vi "Stop Data Logging Session.vi"(8 "error in (no error)":errorcluster, 9 "Clear Session (T)":bool=TRUE, 10 "Session Name in":string, 11 "Data Logging Manager Ref in":T1) -> (0 "error out":errorcluster, 1 "Log File Paths":path[](array[path]), 2 "Session Name out":string, 3 "Data Logging Manager Ref out":T1)   [LabVIEW 2020, in "NI_VS Data Logging API.lvlib"]
doc: "Stops the data logging session specified by <B>Session Name in</B> and returns the paths to all log files generated during the session. This VI attempts to stop the data logging session regardless of any incoming errors."
uses:
  <vilib>/NI VeriStand/Execution/DataLogging/NI_VS Data Logging API.lvlib
  <vilib>/NI VeriStand/Execution/DataLogging/IDataLogging Ref.ctl
  NationalInstruments.VeriStand.ClientAPI
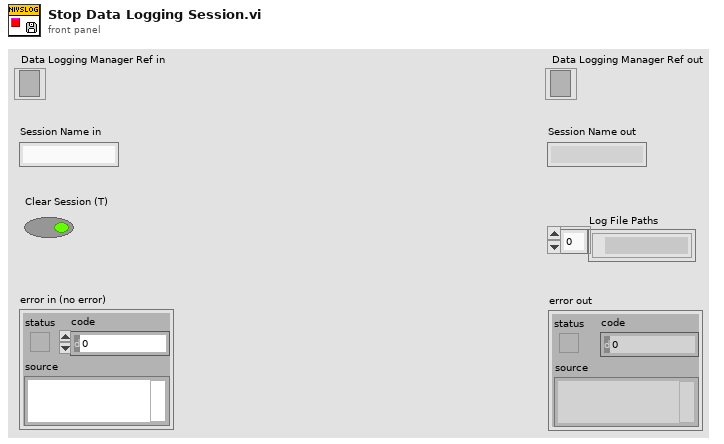
[diagram p1: front panel]
types:
  T1 = typedef "NI_VS Data Logging API.lvlib/IDataLogging Ref.ctl" = refnum<k24>
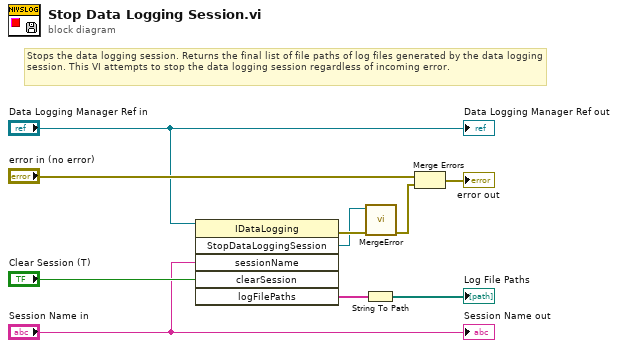
[diagram p0: block diagram]
diagram:
  # "Stops the data logging session. Returns the final list of file paths of log files generated by the data logging session. This VI attempts to stop the data logging session regardless of incoming error."
  n1 = invoke class="IDataLogging" method="StopDataLoggingSession"(reference="Data Logging Manager Ref in", "sessionName"="Session Name in", "clearSession"="Clear Session (T)") -> (error out=w8:errorcluster, "StopDataLoggingSession"=w7:refnum<k24>, "logFilePaths"=w3:string[])  [unwired: 3 in, 3 out]
  n2 = String To Path(string=w3) -> (path=→"Log File Paths":path[])
  n3 = call <vilib>:"MergeError.vi"("error in (no error)"=w8, "Error"=w7) -> ("error out"=w10:errorcluster)  [unwired: 9 out]
  n4 = Merge Errors("error in (no error)", w10) -> (→"error out":errorcluster)
  "Data Logging Manager Ref out" <- "Data Logging Manager Ref in"
  "Session Name out" <- "Session Name in"
